vi "Meas Proc QWTB String to Table Writter.vi"(7 "param table ref":refnum<vi>, 8 "error in":errorcluster, 9 "force data update? (False)":bool, 10 "signaling update? (True)":bool=TRUE, 11 "content csv string":string) -> (0 "error out":errorcluster, 3 "row header changed?":bool)   [LabVIEW 2018]
doc: "This VI will take spreadsheet string table and writes it to the referenced table. It sets formats if the table headers to bold."
uses:
  <vilib>/Utility/miscctls.llb/LVRowAndColumnTypeDef.ctl
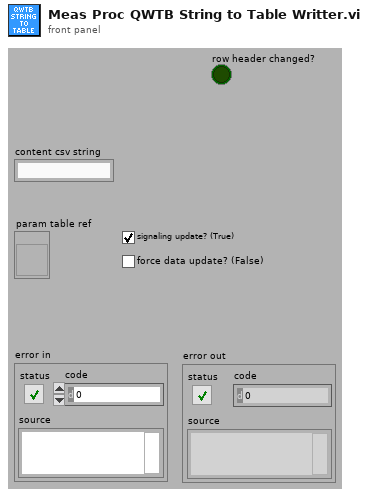
[diagram p1: front panel]
types:
  T1 = typedef "LVRowAndColumnTypeDef.ctl" = cluster{"Row":i32, "Column":i32}
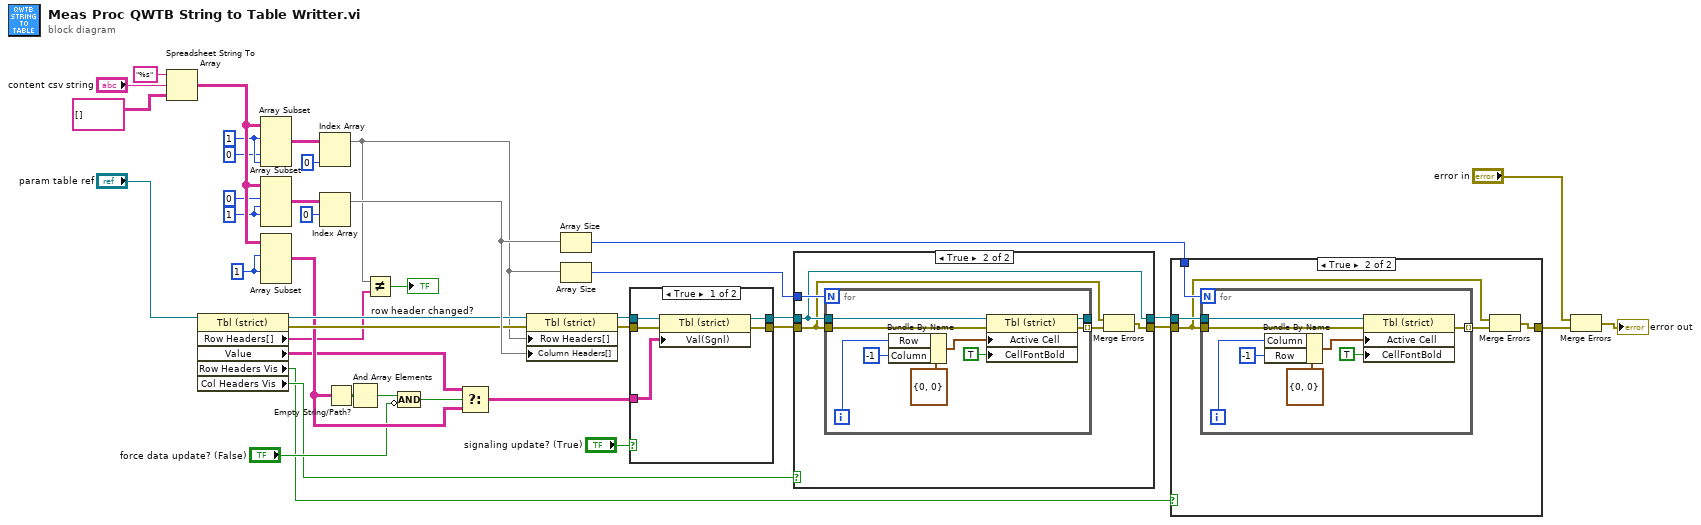
[diagram p0: block diagram]
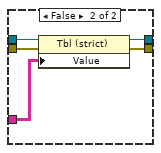
[diagram p4: hidden frame]
diagram:
  w28 = 1 ("index")
  w29 = 1 ("index")
  w24 = 1 ("disabled index (col)")
  n1 = Spreadsheet String To Array(format string="%s", spreadsheet string="content csv string", array type (2D Dbl)=string[][] []) -> (array=w39:string[][])  [unwired: 1 in]
  n2 = property class="Tbl (strict)"(reference="param table ref") -> (reference out=w19:refnum<vi>, error out=w21:errorcluster, "Row Headers[]"=w3:string[], "Value"=w16:string[][], "Row Headers Vis"=w4:bool, "Col Headers Vis"=w5:bool)  [unwired: 1 in]
  n3 = Array Subset(array=w39, index (row)=w28, index (col)=0 ("index"), length (col)=w28) -> (w34:string[][])  [unwired: 1 in]
  n4 = Array Subset(array=w39, index (row)=0 ("disabled index (col)"), length (row)=w24, index (col)=w24) -> (w32:string[][])  [unwired: 1 in]
  n5 = Array Subset(array=w39, index (row)=w29, index (col)=w29) -> (w17:string[][])  [unwired: 2 in]
  n6 = Index Array(array=w34, index (col)=0 ("disabled index (col)")) -> (element=w2:string[])  [unwired: 1 in]
  n7 = Index Array(array=w32, index (row)=0) -> (element=w25:string[])  [unwired: 1 in]
  n8 = Empty String/Path?(string/path=w17) -> (empty?=w18:bool[][])
  n9 = And Array Elements(Boolean array=w18) -> (logical AND=w7:bool)
  n10 = Not Equal?(x=w2, y=w3) -> (x != y?=→"row header changed?":bool)
  n11 = Compound Arithmetic op=AND(w7, invert "force data update? (False)") -> (w8:bool)
  n12 = Select(t=w16, s=w8, f=w17) -> (s? t:f=w10:string[][])
  n13 = property class="Tbl (strict)"(reference=w19, error in=w21, "Row Headers[]"=w2, "Column Headers[]"=w25) -> (reference out=w11:refnum<vi>, error out=w14:errorcluster)
  n14 = Array Size(array=w25) -> (size(s)=w31:i32)
  n15 = Array Size(array=w2) -> (size(s)=w33:i32)
  n16 = case shown="True" "signaling update? (True)" {
    tunnel: w14 -> [w46 w51]
    tunnel: [w45 w50] -> w13
    tunnel: [w44 w49] -> w12
    tunnel: w11 -> [w43 w48]
    tunnel: w10 -> [w42 w47]
    frame True {
      n17 = property class="Tbl (strict)"(reference=w43, error in=w46, "Val(Sgnl)"=w42) -> (reference out=w44:refnum<vi>, error out=w45:errorcluster)
    }
    frame False {
      n18 = property class="Tbl (strict)"(reference=w48, error in=w51, "Value"=w47) -> (reference out=w49:refnum<vi>, error out=w50:errorcluster)
    }
  }
  n19 = case shown="True" w5 {
    tunnel: [w53 w57] -> w37
    tunnel: [w52 w55] -> w36
    tunnel: w33 -> [_ w56]
    tunnel: w13 -> [w53 w54]
    tunnel: w12 -> [w52 w55]
    frame False {
    }
    frame True {
      n20 = for {
        N: w56 -> [_]
        tunnel: w54 -> [w67]
        tunnel: [w61] -> w58 mode=indexing
        tunnel: w55 -> [w60]
        tunnel: [w59] -> _
        i -> [w63]
        n21 = Bundle By Name(cluster=T1 {"Row"=0, "Column"=0} ("Active Cell:Active Cell"), "Row"=w63, "Column"=-1) -> (w66:T1)
        n22 = property class="Tbl (strict)"(reference=w60, error in=w67, "Active Cell"=w66, "CellFontBold"=TRUE ("Active Cell:Cell Font:Bold")) -> (reference out=w59:refnum<vi>, error out=w61:errorcluster)
      }
      n23 = Merge Errors(w54, w58) -> (w57:errorcluster)
    }
  }
  n24 = case shown="True" w4 {
    tunnel: [w68 w70] -> w38
    tunnel: w37 -> [w68 w69]
    tunnel: w36 -> [_ w72]
    tunnel: w31 -> [_ w71]
    frame False {
    }
    frame True {
      n25 = for {
        N: w71 -> [_]
        tunnel: w69 -> [w81]
        tunnel: [w75] -> w73 mode=indexing
        tunnel: w72 -> [w74]
        i -> [w77]
        n26 = Bundle By Name(cluster=T1 {"Row"=0, "Column"=0} ("Active Cell:Active Cell"), "Column"=w77, "Row"=-1 ("Column")) -> (w80:T1)
        n27 = property class="Tbl (strict)"(reference=w74, error in=w81, "Active Cell"=w80, "CellFontBold"=TRUE ("Active Cell:Cell Font:Bold")) -> (error out=w75:errorcluster)  [unwired: 1 out]
      }
      n28 = Merge Errors(w69, w73) -> (w70:errorcluster)
    }
  }
  n29 = Merge Errors("error in", w38) -> (→"error out":errorcluster)
